vi "RouteGuide ListFeatures.vi"(3 "error in (no error)":errorcluster, 4 "gRPCid in":T1, 5 "DNL_LabVIEW Object in":refnum<class "RouteGuideImpl.lvclass">) -> (0 "error out":errorcluster, 1 "gRPCid out":T1, 2 "DNL_LabVIEW Object out":refnum<class "RouteGuideImpl.lvclass">)   [LabVIEW 2019, in "UserCode_server.lvlib" / "RouteGuideImpl.lvclass"]
uses:
  RouteGuideImpl.lvclass
  <vilib>/gRPC/LabVIEW gRPC Library/Shared/grpcId.ctl
  Generated_server/RPC Messages/routeguide_Point.ctl
  Generated_server/Generated_server.lvlib
  Generated_server/RPC Service/RouteGuide/RouteGuide.lvclass
  <vilib>/gRPC/LabVIEW gRPC Library/grpc-lvsupport-release.lvlib
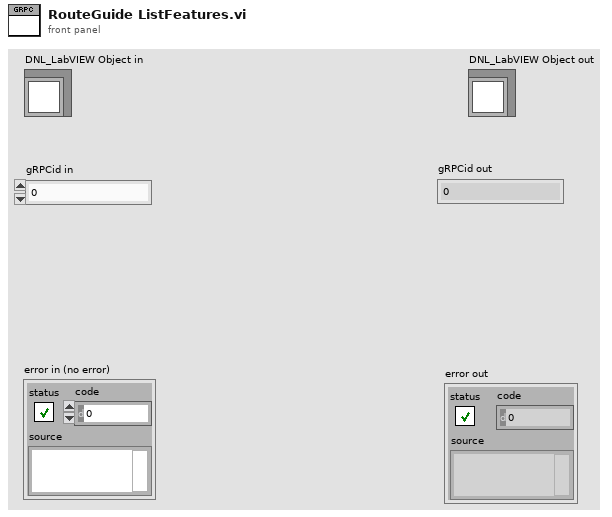
[diagram p1: front panel]
types:
  T1 = typedef "grpc-lvsupport-release.lvlib/grpcId.ctl" = u64
  T2 = typedef "Generated_server.lvlib/routeguide_Point.ctl" = cluster{"latitude":i32, "longitude":i32}
  T3 = typedef "Generated_server.lvlib/routeguide_Rectangle.ctl" = cluster{"lo":T2, "hi":T2}
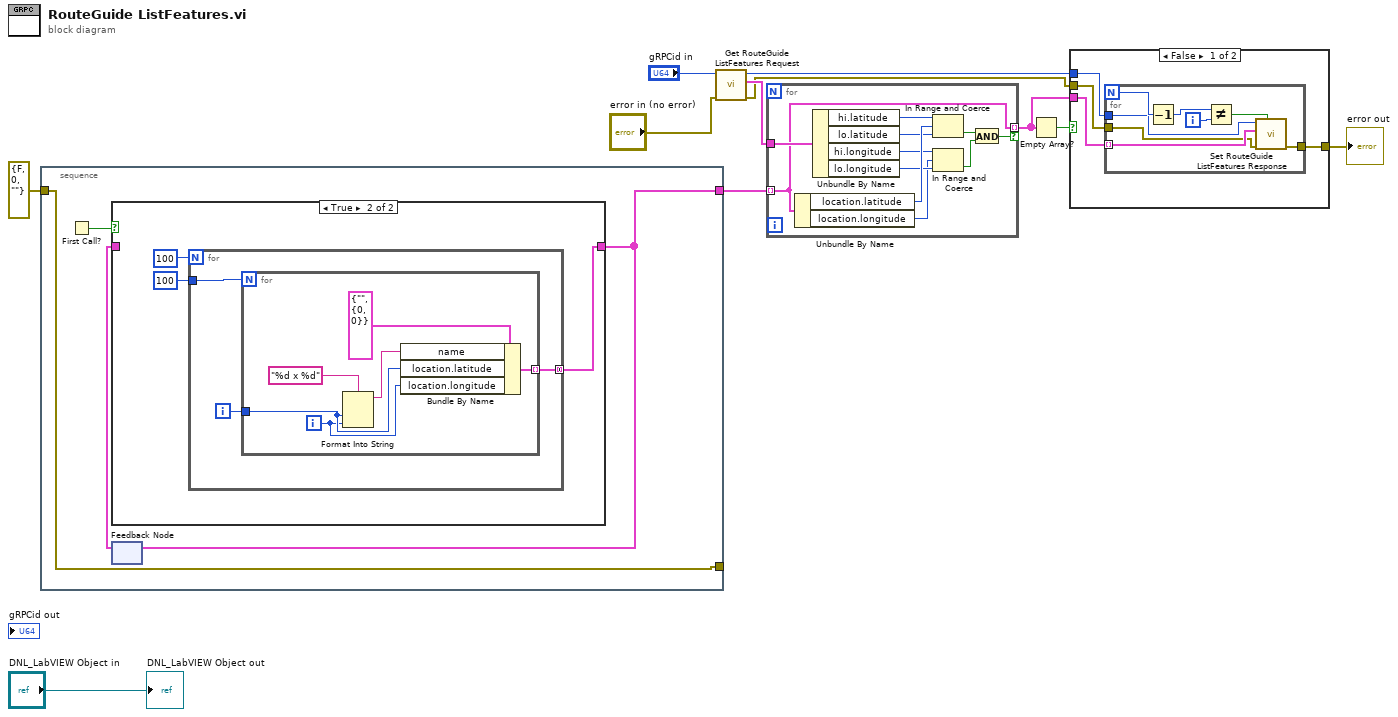
[diagram p0: block diagram]
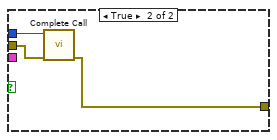
[diagram p3: hidden frame]
diagram:
  n1 = stacked-sequence {
    tunnel: [w12] -> _
    tunnel: [w14] -> w11
    tunnel: errorcluster {"status"=FALSE, "code"=0, "source"=""} ("error in") -> [w12]
    frame #0 {
      n2 = First Call?() -> (First Call?: T/F=w13:bool)
      n3 = feedback #1() -> (w15:cluster{"name":string, "location":T2}[])  [unwired: 1 in]
      n4 = case shown="True" w13 {
        tunnel: [w16 w18] -> w14
        tunnel: w15 -> [w16 _]
        frame False {
        }
        frame True {
          n5 = for {
            N: 100 -> [_]
            tunnel: [w21] -> w18 mode=concatenating
            tunnel: 100 -> [w20]
            i -> [w22]
            n6 = for {
              N: w20 -> [_]
              tunnel: w22 -> [w25]
              tunnel: [w23] -> w21 mode=indexing
              i -> [w24]
              n7 = Format Into String(format string="%d x %d", w25, w24) -> (resulting string=w26:string)  [unwired: 2 in, 1 out]
              n8 = Bundle By Name(cluster=cluster{"name":string, "location":T2} {"name"="", "location"={"latitude"=0, "longitude"=0}} ("routeguide_Feature"), "name"=w26, "location.latitude"=w25, "location.longitude"=w24) -> (w23:cluster{"name":string, "location":T2})
            }
          }
        }
      }
      n9 = feedback-in #1(w14) -> ()
    }
  }
  n10 = call "Get RouteGuide ListFeatures Request.vi"("error in (no error)"="error in (no error)", "gRPCid"="gRPCid in") -> ("error out"=w5:errorcluster, "Message Data"=w6:T3, "gRPCid out"=w7:T1)  [unwired: 7 in]
  n11 = for {
    tunnel: w11 -> [w30] mode=indexing
    tunnel: w6 -> [w39]
    tunnel: [w30] -> w9 mode=indexing if=w29
    n12 = Unbundle By Name(w30) -> ("location.latitude"=w38:i32, "location.longitude"=w33:i32)
    n13 = Unbundle By Name(w39) -> ("hi.latitude"=w37:i32, "lo.latitude"=w36:i32, "hi.longitude"=w35:i32, "lo.longitude"=w34:i32)
    n14 = In Range and Coerce(upper limit=w37, x=w38, lower limit=w36) -> (In Range?=w31:bool)  [unwired: 1 out]
    n15 = In Range and Coerce(upper limit=w35, x=w33, lower limit=w34) -> (In Range?=w32:bool)  [unwired: 1 out]
    n16 = And(x=w31, y=w32) -> (x .and. y?=w29:bool)
  }
  n17 = Empty Array?(array=w9) -> (empty?=w10:bool)
  n18 = case shown="False" w10 {
    tunnel: w7 -> [w43 w53]
    tunnel: w5 -> [w42 w54]
    tunnel: w9 -> [w41 _]
    tunnel: [w40 w52] -> w1
    frame False {
      n19 = for {
        N -> [w51]
        tunnel: w43 -> [w47]
        tunnel: w42 -> [w45]
        tunnel: w41 -> [w46] mode=indexing
        tunnel: [w44] -> w40
        i -> [w50]
        n20 = Decrement(x=w51) -> (x-1=w49:i32)
        n21 = Not Equal?(x=w49, y=w50) -> (x != y?=w48:bool)
        n22 = call "Set RouteGuide ListFeatures Response.vi"("Streaming? (F)"=w48, "error in (no error)"=w45, "Message Data"=w46, "gRPCid in"=w47) -> ("error out"=w44:errorcluster)  [unwired: 7 in]
      }
    }
    frame True {
      n23 = call <vilib>:"Complete Call.vi"("gRPCid"=w53, "error in"=w54) -> ("error out"=w52:errorcluster)  [unwired: 8 in]
    }
  }
  "error out" <- w1
  "DNL_LabVIEW Object out" <- "DNL_LabVIEW Object in"
